vi "Decode IP Packet.vi"(11 "IP Packet":u8[](array[numeric]) format="%02x") -> (2 "Data Out":u8[](array[numeric]) format="%02x", 3 "IP Packet":T1 {"Header Checksum" format="%04x"; "Flags" format="%02x"; "Type of Service" format="%02x"})   [LabVIEW 2018]
uses:
  IP Packet Info.ctl
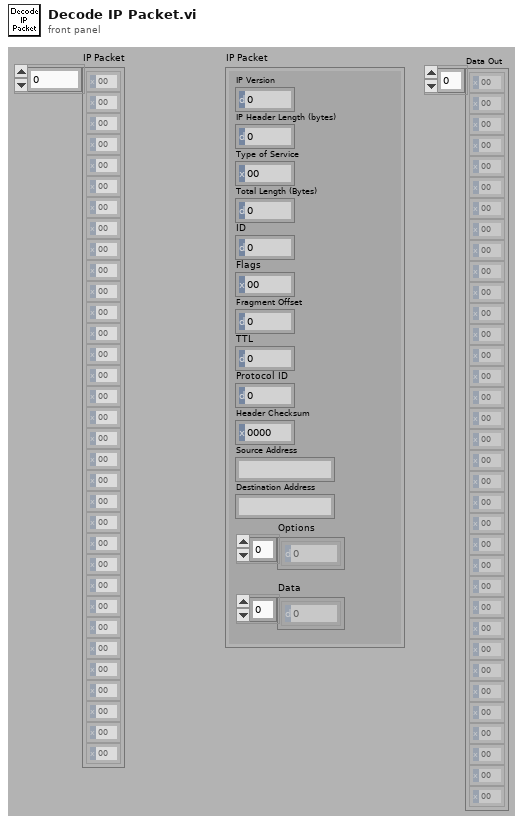
[diagram p1: front panel]
types:
  T1 = typedef "IP Packet Info.ctl" = cluster{"IP Version":u8, "IP Header Length (bytes)":u8, "Type of Service":u8, "ID":u16, "Flags":u8, "Total Length (Bytes)":u16, "Fragment Offset":u16, "TTL":u8, "Protocol ID":u8, "Header Checksum":u16, "Source Address":string, "Destination Address":string, "Options":u8[], "Data":u8[]}
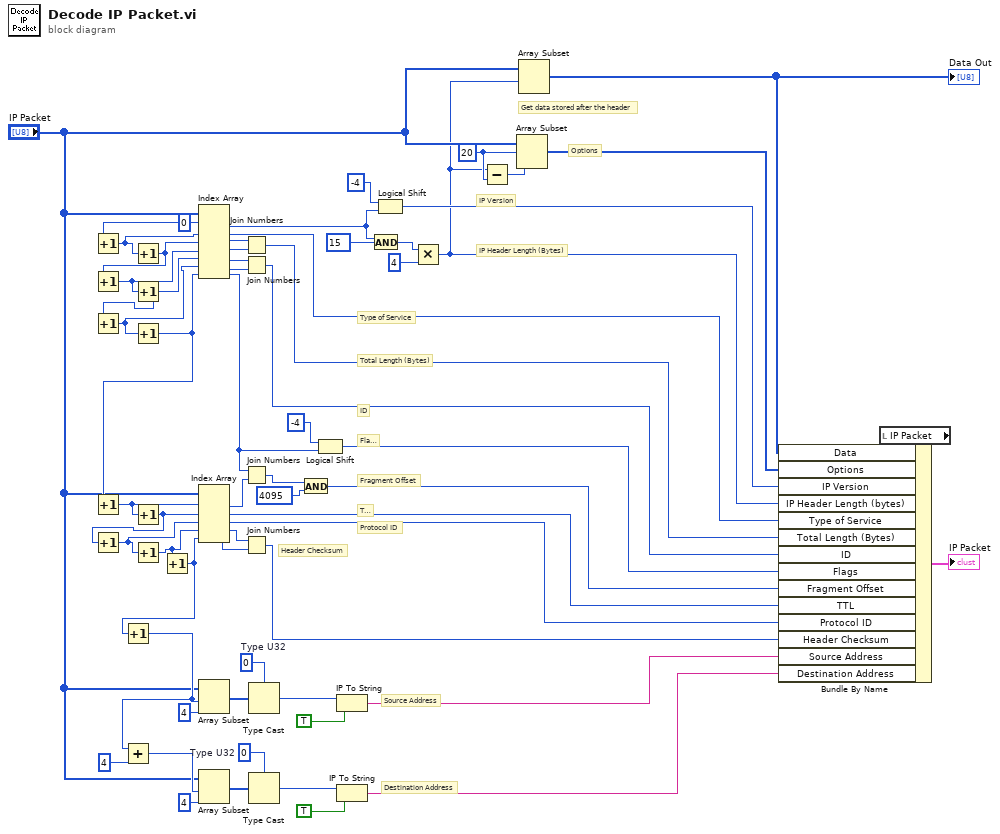
[diagram p0: block diagram]
diagram:
  w7 = 20 ("index")
  w2 = u32 0  # Type U32
  w1 = u32 0  # Type U32
  w45 = 0 ("index")
  # "Get data stored after the header"
  # "IP Version"
  # "IP Header Length (Bytes)"
  # "Type of Service"
  # "Total Length (Bytes)"
  # "ID"
  # "Flags"
  # "Fragment Offset"
  # "TTL"
  # "Protocol ID"
  # "Header Checksum"
  # "Source Address"
  # "Destination Address"
  # "Options"
  n1 = Increment(x=w45) -> (x+1=w44:i32)
  n2 = Increment(x=w44) -> (x+1=w43:i32)
  n3 = Increment(x=w43) -> (x+1=w42:i32)
  n4 = Increment(x=w42) -> (x+1=w41:i32)
  n5 = Increment(x=w41) -> (x+1=w40:i32)
  n6 = Increment(x=w40) -> (x+1=w39:i32)
  n7 = Increment(x=w39) -> (x+1=w51:i32)
  n8 = Increment(x=w51) -> (x+1=w50:i32)
  n9 = Increment(x=w50) -> (x+1=w49:i32)
  n10 = Increment(x=w49) -> (x+1=w48:i32)
  n11 = Increment(x=w48) -> (x+1=w37:i32)
  n12 = Increment(x=w37) -> (x+1=w29:i32)
  n13 = Add(x=w29, y=4) -> (x+y=w22:i32)
  n14 = Index Array(array="IP Packet", index #1=w45, index #2=w44, index #3=w43, index #4=w42, index #5=w41, index #6=w40, index #7=w39) -> (element #1=w59:u8, element #2=w18:u8, element #3=w55:u8, element #4=w54:u8, element #5=w53:u8, element #6=w52:u8, element #7=w26:u8)
  n15 = Index Array(array="IP Packet", index #1=w51, index #2=w50, index #3=w49, index #4=w48, index #5=w37) -> (element #1=w25:u8, element #2=w13:u8, element #3=w12:u8, element #4=w47:u8, element #5=w46:u8)
  n16 = Array Subset(array="IP Packet", index=w29, length=4) -> (w38:u8[])
  n17 = Array Subset(array="IP Packet", index=w22, length=4) -> (w30:u8[])
  n18 = Join Numbers(hi=w55, lo=w54) -> ((hi.lo)=w17:u16)
  n19 = Join Numbers(hi=w53, lo=w52) -> ((hi.lo)=w16:u16)
  n20 = Join Numbers(hi=w26, lo=w25) -> ((hi.lo)=w24:u16)
  n21 = Join Numbers(hi=w47, lo=w46) -> ((hi.lo)=w11:u16)
  n22 = Type Cast(type=w1, x=w38) -> (*(type *) &x=w35:u32)
  n23 = Type Cast(type=w2, x=w30) -> (*(type *) &x=w32:u32)
  n24 = And(x=w24, y=u16 4095) -> (x .and. y?=w14:u16)
  n25 = Logical Shift(y=-4, x=w26) -> (x << y=w15:u8)
  n26 = IP To String(1:TRUE ("dot notation? (F)"), 2:w35) -> (0:w10:string)
  n27 = IP To String(1:TRUE ("dot notation? (F)"), 2:w32) -> (0:w9:string)
  n28 = And(x=w59, y=u8 15) -> (x .and. y?=w57:u8)
  n29 = Logical Shift(y=-4, x=w59) -> (x << y=w19:u8)
  n30 = Multiply(x=w57, y=u8 4) -> (x*y=w4:u8)
  n31 = Subtract(x=w4, y=w7) -> (x-y=w8:i32)
  n32 = Array Subset(array="IP Packet", index=w7, length=w8) -> (w6:u8[])
  n33 = Array Subset(array="IP Packet", index=w4) -> (w3:u8[])  [unwired: 1 in]
  "Data Out" <- w3
  n34 = local read "IP Packet"() -> (w21:T1)
  n35 = Bundle By Name(cluster=w21, "Data"=w3, "Options"=w6, "IP Version"=w19, "IP Header Length (bytes)"=w4, "Type of Service"=w18, "Total Length (Bytes)"=w17, "ID"=w16, "Flags"=w15, "Fragment Offset"=w14, "TTL"=w13, "Protocol ID"=w12, "Header Checksum"=w11, "Source Address"=w10, "Destination Address"=w9) -> (→"IP Packet":T1)
